vi "Channel Name.vi"(8 "error in (no error)":errorcluster, 11 "Scale in":refnum<class "Scale Config.lvclass">) -> (0 "error out":errorcluster, 1 "Is Channel":bool, 2 "Channel Name":string, 3 "Scale out":refnum<class "Scale Config.lvclass">)   [LabVIEW 2023, in "VolatusConfig.lvlib" / "Scale Config.lvclass"]
uses:
  Scale Config.lvclass
  C:/dev/volatus/mts-volatus-super/libs/lv-volatus/VolatusConfig/VolatusConfigElement/VolatusConfigElement.lvclass
  Meta Type.ctl
  VolatusConfigElement/VolatusConfigElement.lvclass/VolatusConfigElement.ctl
  VolatusConfigElement/Element.vi
  lv-cdm/CDM-Config/Config Lookup/Match Meta.vi
  lv-cdm/CDM-Config/Config Element/Owner.vi
  lv-cdm/CDM-Config/Config Filter/Config Lookup.lvclass
  Scale Config.lvclass/Scale Config.ctl
  VolatusConfigElement/VolatusConfigElement.lvclass
  VolatusConfig.lvlib
  lv-cdm/CDM-Config/Config Element/Config Element.lvclass
  C:/dev/volatus/mts-volatus-super/libs/lv-volatus/VolatusConfig/Scale/Scale Config.lvclass
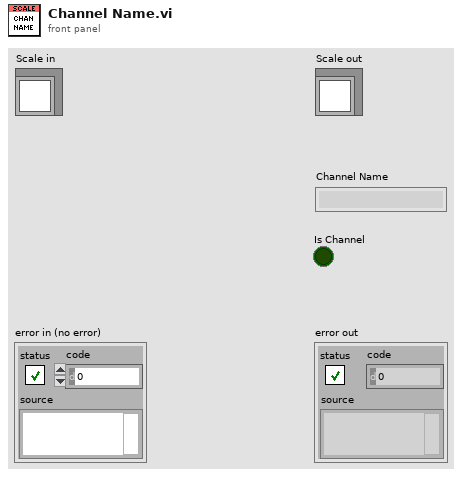
[diagram p1: front panel]
types:
  T1 = typedef "VolatusConfig.lvlib/Meta Type.ctl" = enum16{"UNKNOWN", "VL_System", "VL_Cluster", "VL_Node", "VL_Task", "VL_Group", "VL_Channel", "VL_Task_List", "VL_Scaling", "VL_Sensor", "VL_Sensor_List", "VL_Scale"}
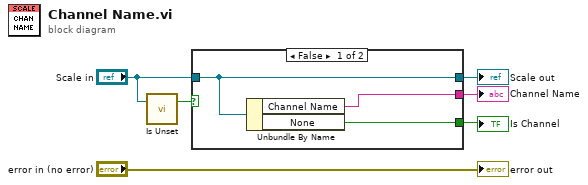
[diagram p0: block diagram]
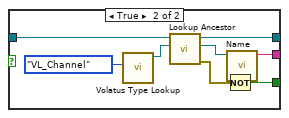
[diagram p2: hidden frame]
diagram:
  n1 = call "Is Unset.vi"("VolatusConfigElement in"="Scale in") -> ("Unset"=w1:bool)  [unwired: 6 in]
  n2 = case shown="False" w1 {
    tunnel: [w7 w17] -> w5
    tunnel: [w8 w13] -> w4
    tunnel: [w9 w11] -> w3
    tunnel: "Scale in" -> [w7 w10]
    frame False {
      n3 = Unbundle By Name(w7) -> ("Channel Name"=w8:string, "None"=w9:bool)
    }
    frame True {
      n4 = call "Volatus Type Lookup.vi"("Meta Type"=Meta_Type."VL_Channel") -> ("Config Lookup out"=w15:refnum<class "Config Lookup.lvclass">)  [unwired: 9 in, 1 out]
      n5 = call "Lookup Ancestor.vi"("Lookup"=w15, "VolatusConfigElement in"=w10) -> ("error out"=w12:errorcluster, "Ancestor"=w14:refnum<class "Config Element.lvclass">, "VolatusConfigElement out"=w17:refnum<class "Scale Config.lvclass">)  [unwired: 7 in]
      n6 = Not(x=w12) -> (.not. x?=w11:bool)
      n7 = call "Name.vi"("Config Element in"=w14) -> ("Name"=w13:string)  [unwired: 9 in, 1 out]
    }
  }
  "Scale out" <- w5
  "Channel Name" <- w4
  "Is Channel" <- w3
  "error out" <- "error in (no error)"
